vi "Load & Verify PFX Certificate.vi"(8 "error in (no error)":errorcluster, 11 "PFX Certificate in":T1) -> (0 "error out":errorcluster, 3 "X509 Certificate out":refnum<k24>)   [LabVIEW 2013, in "dotNET SSL Socket.lvlib" / "dotNET SSL Socket.lvclass"]
doc: "Loads a PFX certificate into a X509 Certificate object and verifies the certificate."
uses:
  dotNET SSL Socket.lvclass
  PFX Certificate.ctl
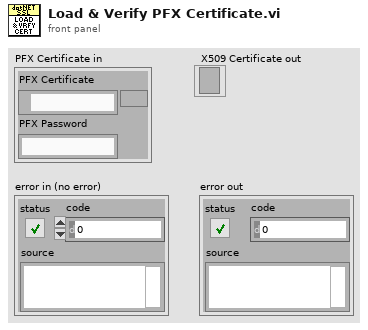
[diagram p1: front panel]
types:
  T1 = typedef "dotNET SSL Socket.lvlib/dotNET SSL Socket.lvclass/PFX Certificate.ctl" = cluster{"PFX Certificate":path, "PFX Password":string}
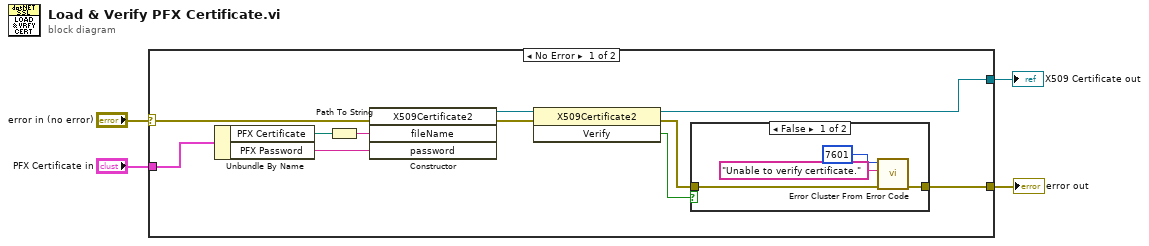
[diagram p0: block diagram]
diagram:
  n1 = case shown="No Error" "error in (no error)" {
    selector: "error in (no error)" -> [w5 w21]
    tunnel: "PFX Certificate in" -> [w13 _]
    tunnel: [w12 _] -> w3
    tunnel: [w11 w21] -> w2
    frame No Error {
      n2 = Unbundle By Name(w13) -> ("PFX Certificate"=w14:path, "PFX Password"=w15:string)
      n3 = Path To String(path=w14) -> (string=w8:string)
      n4 = constructor class="X509Certificate2"(error in=w5, "fileName"=w8, "password"=w15) -> (reference out=w6:refnum<k24>, error out=w7:errorcluster)  [unwired: 2 in, 3 out]
      n5 = invoke class="X509Certificate2" method="Verify"(reference=w6, error in=w7) -> (reference out=w12:refnum<k24>, error out=w10:errorcluster, "Verify"=w9:bool)  [unwired: 1 in]
      n6 = case shown="False" w9 {
        tunnel: w10 -> [w18 w20]
        tunnel: [w19 w20] -> w11
        frame False {
          n7 = call <vilib>:"Error Cluster From Error Code.vi"("error in (no error)"=w18, "error message (\"\")"="Unable to verify certificate." ("error message (\"\")"), "error code (0)"=7601) -> ("error out"=w19:errorcluster)  [unwired: 6 in]
        }
        frame True {
        }
      }
    }
    frame Error {
    }
  }
  "X509 Certificate out" <- w3
  "error out" <- w2
